vi "Get Current Speed.vi"(8 "error in (no error)":errorcluster, 11 "Fine SIM Motion Controller in":refnum<class "Fine SIM Motion Controller.lvclass">) -> (0 "error out":errorcluster, 2 "Current Speed":dbl, 3 "Fine SIM Motion Controller out":refnum<class "Fine SIM Motion Controller.lvclass">)   [LabVIEW 2022 SP3, in "Fine SIM Motion Controller.lvclass"]
uses:
  Fine SIM Motion Controller.lvclass
  Fine SIM Motion Controller.lvclass/Fine SIM Motion Controller.ctl
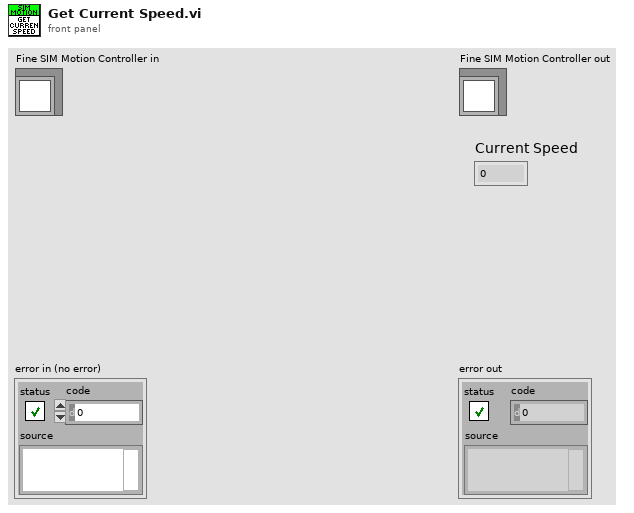
[diagram p1: front panel]
types:
  T1 = typedef "Parent SIM Motion Controller.lvclass/Axis Data.ctl" = cluster{"Axis Parameters":T2, "Axis Settings":T4, "Time Stamp":timestamp}
  T2 = typedef "Parent SIM Motion Controller.lvclass/Axis Parameters.ctl" = cluster{"Moving":bool, "Homed":bool, "Desired Position":dbl, "Current Positon":dbl, "Current Speed":dbl, "Home Status":T3}
  T3 = typedef "Parent SIM Motion Controller.lvclass/Homing Status.ctl" = enum16{"Idle", "Inital Home Motion", "Final Home Motion", "Done Homing"}
  T4 = typedef "Parent SIM Motion Controller.lvclass/Axis Settings.ctl" = cluster{"Speed":dbl, "Acceleration":dbl}
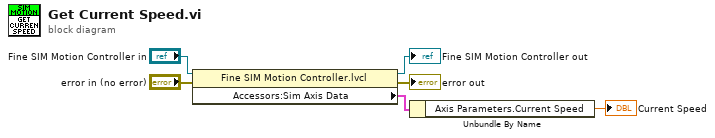
[diagram p0: block diagram]
diagram:
  n1 = property class="Fine SIM Motion Controller.lvcl"(reference="Fine SIM Motion Controller in", error in="error in (no error)") -> (reference out=→"Fine SIM Motion Controller out":refnum<class "Fine SIM Motion Controller.lvclass">, error out=→"error out":errorcluster, "Accessors:Sim Axis Data"=w4:T1)
  n2 = Unbundle By Name(w4) -> ("Axis Parameters.Current Speed"=→"Current Speed":dbl)
